vi "Arydh engine fronend.vi"   [LabVIEW 2018]
uses:
  publisher action.ctl
  Users/Nanocal/Desktop/Calorimetry v1.3/MCL.lvlibp
panel:
  # "Engine frontend"
types:
  T1 = typedef "publisher action.ctl" = enum16{"set", "get", "init", "check"}
  T2 = typedef "MCL.lvlibp/MCL_DataRef.ctl" = refnum<vi>
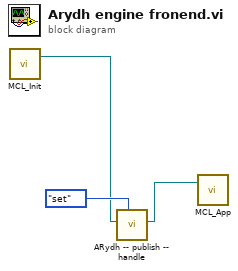
[diagram p0: block diagram]
diagram:
  n1 = call "MCL_Init.vi"() -> ("MCL object"=w1:T2)  [unwired: 2 in, 1 out]
  n2 = call "ARydh -- publish -- handle.vi"("publisher action"=publisher_action."set", "MCL object"=w1) -> ("MCL object OUT"=w2:T2)  [unwired: 9 in]
  n3 = call "MCL_App.vi"("MCL object"=w2) -> ()  [unwired: 3 in]
